vi "DMR_ImageRequestUnlock.vi"(4 "request number IN":i32, 5 "driver handle IN":i32) -> (0 "error code OUT":i32, 2 "driver handle OUT":i32)   [LabVIEW 2016]
doc: "Unlocks the request for the driver again.\n\nTo ensure that no image data is overwritten by another image request while the user still deals with the image from a previous acquisition each image buffer will be locked by the driver when it is returned to the user by a call to DMR_ImageRequestWaitFor.\n\nNo new image will be captured into the same buffer until the user unlocks the buffer again by calling DMR_ImageRequestUnlock.\n\nSee also:\nDMR_ImageRequestReset,\nDMR_ImageRequestSingle,\nDMR_ImageRequestWaitFor\n\nThe 'error code OUT' terminal will deliver 0 if successful or a negative error code otherwise. A list of valid error codes and their meaning can be found in the manual about this interface."
uses:
  mvDeviceManager.dll
panel:
  # "OUTPUT"
  # "INPUT"
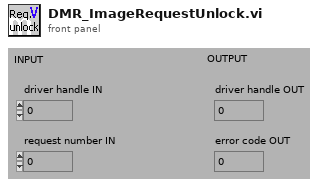
[diagram p1: front panel]
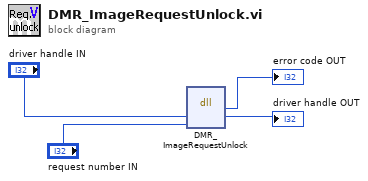
[diagram p0: block diagram]
diagram:
  n1 = dll-call lib="mvDeviceManager.dll" fn="DMR_ImageRequestUnlock"("hDrv"="driver handle IN", "requestNr"="request number IN") -> (→"error code OUT":i32, "hDrv"=→"driver handle OUT":i32)  [unwired: 4 in, 2 out]
